vi "Wait for Edge.vi"(0 "Clk":refnum<k21>="Port8/DIOCTL", 5 "Falling Edge":bool, 11 "Error IN":errorcluster) -> (15 "Error OUT":errorcluster)   [LabVIEW 2011]
uses:
  <vilib>/rvi/eio/common/nirviEmuTemplateMethod_errors.vi
  <vilib>/eio/EIONode/EIONode.xnode
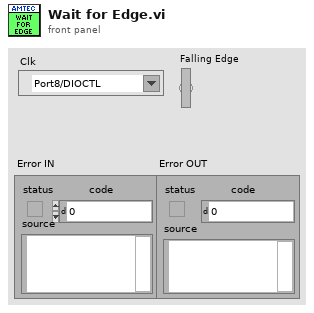
[diagram p1: front panel]
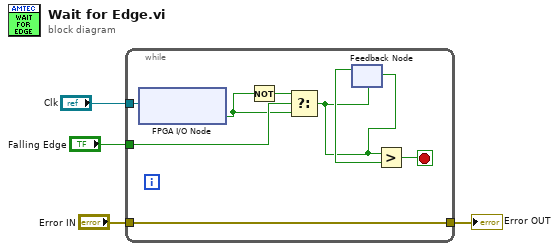
[diagram p0: block diagram]
diagram:
  n1 = while {
    tunnel: "Clk" -> [w6]
    tunnel: [w11] -> w3
    tunnel: "Error IN" -> [w11]
    tunnel: "Falling Edge" -> [w7]
    stop <- w9 stop-if-true
    n2 = xnode "FPGA I/O Node"("FPGA I/O In"=w6) -> ("I/O Item"=w5:bool)  [unwired: 1 out]
    n3 = Not(x=w5) -> (.not. x?=w12:bool)
    n4 = Select(t=w12, s=w7, f=w5) -> (s? t:f=w8:bool)
    n5 = feedback-in #1(w8) -> ()
    n6 = feedback #1(w8) -> (w10:bool)
    n7 = Greater?(x=w8, y=w10) -> (0:w9:bool)
  }
  "Error OUT" <- w3
